vi "Test Initialize.vi"(8 "error in (no error)":errorcluster) -> (0 "error out":errorcluster, 3 "body":string)   [LabVIEW 2020, in "MCP Server tests.lvlib"]
uses:
  MCP Server tests.lvlib
  <vilib>/JDP Science/JSONtext/Next JSON Value.vi
  <vilib>/JDP Science/JSONtext/String Subset.vi
  <vilib>/JDP Science/JSONtext/Parsing/Advance past next JSON Value (inlined COPY).vi
  <vilib>/JDP Science/JSONtext/Parsing/Advance past whitespace.vi
  <vilib>/JDP Science/JSONtext/Parsing/Advance past String.vi
  <vilib>/JDP Science/JSONtext/Parsing/Advance past Number.vi
  <vilib>/JDP Science/JSONtext/Parsing/Advance past Line Ending.vi
  <vilib>/JDP Science/JSONtext/Parsing/Parse Full Path or Item Name.vi
  <vilib>/JDP Science/JSONtext/Parsing/Advance past Array.vi
  <vilib>/JDP Science/JSONtext/Parsing/Advance past Object.vi
  <vilib>/JDP Science/JSONtext/support/Error Cluster From Code.vi
  <vilib>/JDP Science/JSONtext/Offset/Find Item Locations by Path.vi
  <vilib>/addons/_JKI Toolkits/Caraya/classes/Test/Test.lvclass
  <vilib>/addons/_JKI Toolkits/Caraya/classes/Assert/Assert.lvclass
  <vilib>/JDP Science/JSONtext/JSONtext.lvlib
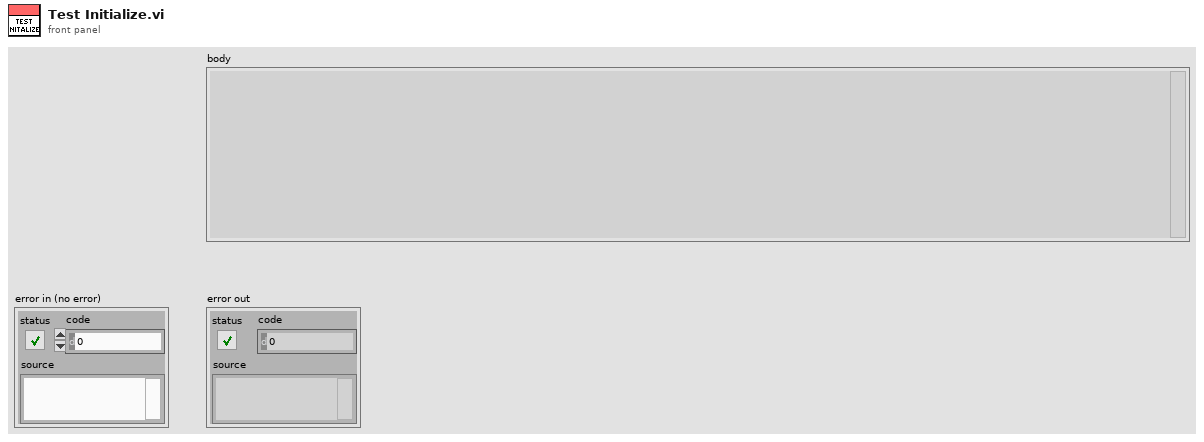
[diagram p1: front panel]
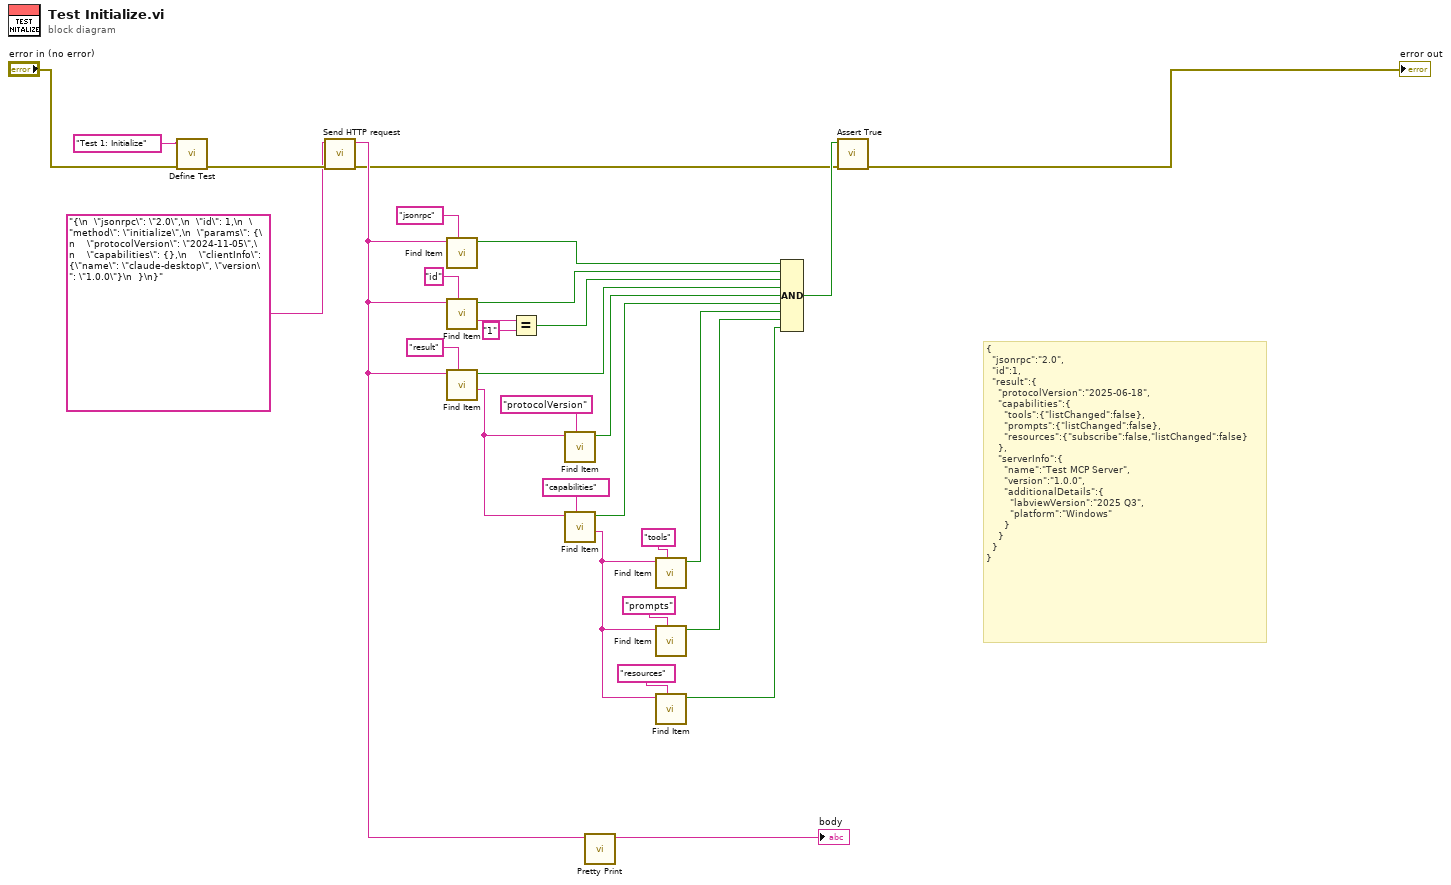
[diagram p0: block diagram]
diagram:
  # "{\n  \"jsonrpc\":\"2.0\",\n  \"id\":1,\n  \"result\":{\n    \"protocolVersion\":\"2025-06-18\",\n    \"capabilities\":{\n      \"tools\":{\"listChanged\":false},\n      \"prompts\":{\"listChanged\":false},\n      \"resources\":{\"subscribe\":false,\"listChanged\":false}\n    },\n    \"serverInfo\":{\n      \"name\":\"Test MCP Server\",\n      \"version\":\"1.0.0\",\n      \"additionalDetails\":{\n        \"labviewVersion\":\"2025 Q3\",\n        \"platform\":\"Windows\"\n      }\n    }\n  }\n}"
  n1 = call <vilib>:"Define Test.vi"("error in (no error)"="error in (no error)", "Label (VI Title)"="Test 1: Initialize") -> ("error out"=w17:errorcluster)  [unwired: 8 in, 1 out]
  n2 = call "Send HTTP request.vi"("error in (no error)"=w17, "request"="{\n  \"jsonrpc\": \"2.0\",\n  \"id\": 1,\n  \"method\": \"initialize\",\n  \"params\": {\n    \"protocolVersion\": \"2024-11-05\",\n    \"capabilities\": {},\n    \"clientInfo\": {\"name\": \"claude-desktop\", \"version\": \"1.0.0\"}\n  }\n}" ("buffer")) -> ("error out"=w18:errorcluster, "response"=w29:string)  [unwired: 7 in, 1 out]
  n3 = call <vilib>:"Find Item.vi"("$Path or Item Name"="jsonrpc", "JSON"=w29) -> ("Found"=w23:bool)  [unwired: 6 in, 3 out]
  n4 = call <vilib>:"Find Item.vi"("$Path or Item Name"="id", "JSON"=w29) -> ("<JSON>"=w21:string, "Found"=w24:bool)  [unwired: 6 in, 2 out]
  n5 = call <vilib>:"Find Item.vi"("$Path or Item Name"="result", "JSON"=w29) -> ("<JSON>"=w9:string, "Found"=w28:bool)  [unwired: 6 in, 2 out]
  n6 = Equal?(x=w21, y="1") -> (x = y?=w25:bool)
  n7 = call <vilib>:"Find Item.vi"("$Path or Item Name"="protocolVersion", "JSON"=w9) -> ("Found"=w11:bool)  [unwired: 6 in, 3 out]
  n8 = call <vilib>:"Find Item.vi"("$Path or Item Name"="capabilities", "JSON"=w9) -> ("<JSON>"=w4:string, "Found"=w8:bool)  [unwired: 6 in, 2 out]
  n9 = call <vilib>:"Pretty Print.vi"("JSON"=w29) -> ("<JSON>"=→"body":string)  [unwired: 8 in, 2 out]
  n10 = call <vilib>:"Find Item.vi"("$Path or Item Name"="tools", "JSON"=w4) -> ("Found"=w3:bool)  [unwired: 6 in, 3 out]
  n11 = call <vilib>:"Find Item.vi"("$Path or Item Name"="prompts", "JSON"=w4) -> ("Found"=w2:bool)  [unwired: 6 in, 3 out]
  n12 = call <vilib>:"Find Item.vi"("$Path or Item Name"="resources", "JSON"=w4) -> ("Found"=w1:bool)  [unwired: 6 in, 3 out]
  n13 = Compound Arithmetic op=AND(w23, w24, w25, w28, w11, w8, w3, w2, w1) -> (w26:bool)
  n14 = call <vilib>:"Assert True.vi"("error in (no error)"=w18, "True?"=w26) -> ("error out"=→"error out":errorcluster)  [unwired: 8 in, 1 out]
